vi "MC5e Global_Error_Codes.vi"() -> ()   [LabVIEW 2020]
panel:
  in  "Credentials Not Valid":errorcluster={"status"=TRUE, "code"=-5020, "source"="P&G Credentials closed or invalid.  Access to the BLISS servers requires valid P&G credentials.\n"}
  in  "Load config XML wrong format":errorcluster={"status"=TRUE, "code"=-5019, "source"="The XML format is invalid.  This may be caused either by attempting to load a config file from an older version or if the xml file was incorrectly edited.\n"}
  in  "Invalid Folder":errorcluster={"status"=TRUE, "code"=-5018, "source"="The Image Save Folder does not exist or insufficient permissions.  You are required to select only existing folders to which you have read and write permissions.  If the folder already exists, then this user or machine may not have write permissions to the selected folder.  Please check the permissions or choose or create another folder.\n"}
  in  "CSV Read Error":errorcluster={"status"=TRUE, "code"=-5017, "source"="The file could not be opened or the file is in the wrong format.  The list of BLISS Servers should be in CSV (comma separated variable) list format.\n"}
  in  "server offline":errorcluster={"status"=TRUE, "code"=-5016, "source"="The server could not be found.  Make sure the sever name is spelled correctly.  Also check that you are on the P&G network or connected to the P&G network via VPN.  Also, you may need to sign in to through the User Authentication Firewall.  \nSee https://uac.pg.com/dana-na/auth/url_1/welcome.cgi\nAs of November 2020, you should use PING to authenticate through the USC Firewalls.\n"}
  in  "empty server index":errorcluster={"status"=TRUE, "code"=-5015, "source"="The none of the server names are blank.  If loading a list of servers from a file, please check the server.csv. There should be no blank or skipped lines and there shold not be an empty line at the end or start of the file.\n"}
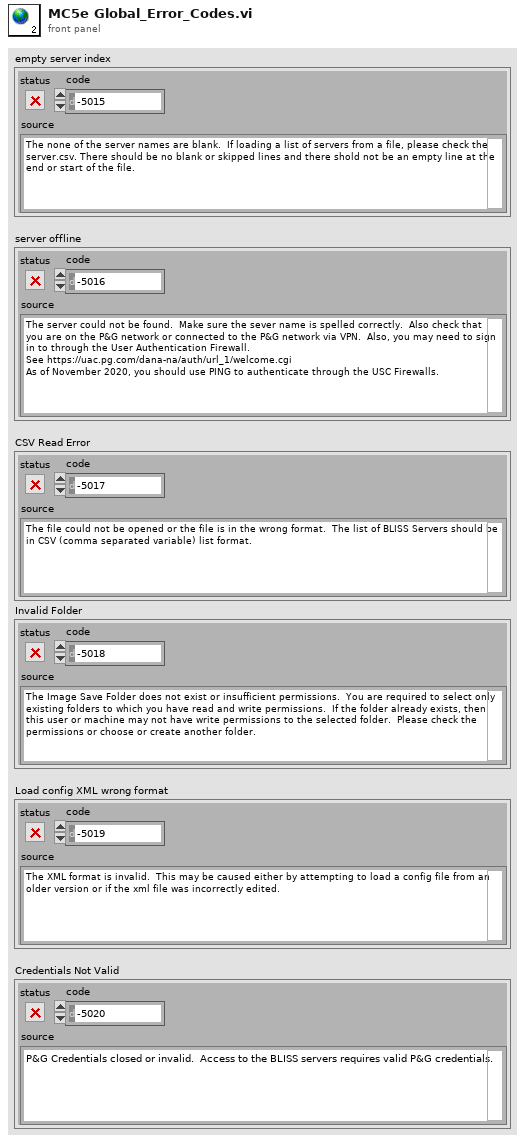
[diagram p1: front panel]
diagram:
